vi "DeadBand.vi"(8 "Deadband":dbl, 11 "Input":dbl) -> (3 "Output":dbl)   [LabVIEW 2020]
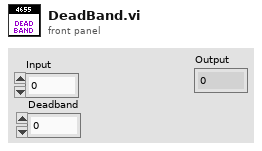
[diagram p1: front panel]
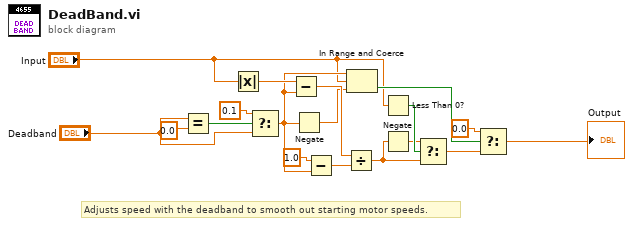
[diagram p0: block diagram]
diagram:
  # "Adjusts speed with the deadband to smooth out starting motor speeds."
  n1 = Equal?(x="Deadband", y=0.0) -> (x = y?=w6:bool)
  n2 = Absolute Value(x="Input") -> (abs(x)=w16:dbl)
  n3 = Select(t=0.1, s=w6, f="Deadband") -> (s? t:f=w7:dbl)
  n4 = Subtract(x=w16, y=w7) -> (x-y=w15:dbl)
  n5 = Negate(x=w7) -> (-x=w10:dbl)
  n6 = Subtract(x=1.0, y=w7) -> (x-y=w8:dbl)
  n7 = Divide(x=w15, y=w8) -> (x/y=w12:dbl)
  n8 = In Range and Coerce(upper limit=w7, x="Input", lower limit=w10) -> (In Range?=w18:bool)  [unwired: 1 out]
  n9 = Less Than 0?(x="Input") -> (x < 0?=w14:bool)
  n10 = Negate(x=w12) -> (-x=w13:dbl)
  n11 = Select(t=w13, s=w14, f=w12) -> (s? t:f=w11:dbl)
  n12 = Select(t=0.0, s=w18, f=w11) -> (s? t:f=→"Output":dbl)
